vi "create default channels.vi"() -> (0 "error out":errorcluster, 1 "names":string[](array[string]), 2 "channels":refnum<class "TBM channel.lvclass">[](array[class]), 3 "module":refnum<class "UI Reference configuration.lvclass">, 5 "instance identifier":string)   [LabVIEW 2013, in "UI reference module tests.lvlib"]
uses:
  UI reference module tests.lvlib
  <vilib>/NI/Tag Bus Module Framework/channel/TBM channel.lvclass
  module/configuration/UI Reference configuration.lvclass
  <vilib>/NI/Tag Bus Module Framework/channel/channel classification.ctl
  module/configuration/UI Reference configuration.lvclass/UI Reference configuration.ctl
  module/configuration/Write VI name.vi
  module/configuration/Write VI Refnum.vi
  <vilib>/NI/Tag Bus Module Framework/root configuration/TBM configuration.lvclass
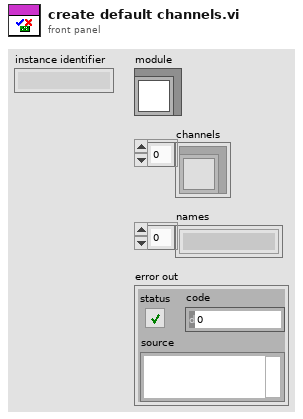
[diagram p1: front panel]
types:
  T1 = typedef "TBM channel.lvclass/channel classification.ctl" = enum16{"input data", "output data", "processing parameter", "processing result"}
  T2 = typedef "tag bus.lvlib/tag descriptor.lvclass/Data Type.ctl" = enum16{"Double", "Single", "I64", "I32", "I16", "I8", "U64", "U32", "U16", "U8", "Boolean", "String", "Array of Double", "Array of Single", "Array of I64", "Array of I32", "Array of I16", "Array of I8", "Array of U64", "Array of U32", "Array of U16", "Array of U8", "Array of Boolean", "Array of String"}
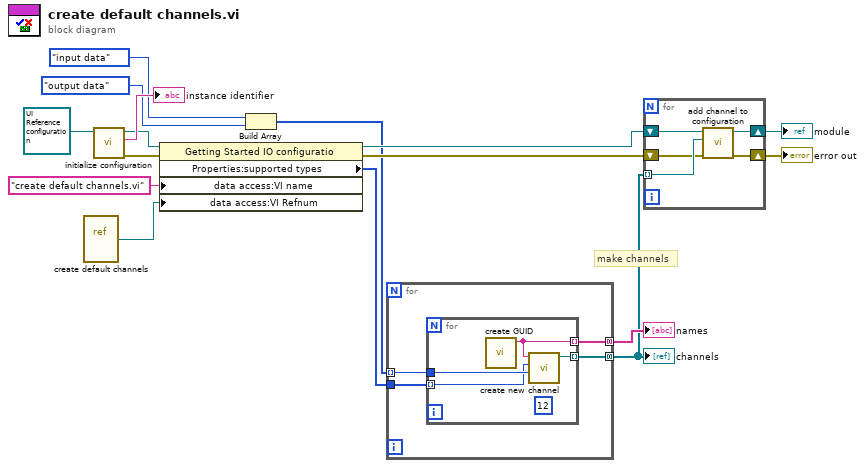
[diagram p0: block diagram]
diagram:
  # "make channels"
  n1 = vi-ref "create default channels.vi"() -> (w1:refnum<vi>)
  n2 = call-dynamic "initialize configuration.vi"("configuration in"=refnum<class "UI Reference configuration.lvclass"> refnum ("tag bus configurable plugin module configuration")) -> ("error out"=w14:errorcluster, "instance identifier"=→"instance identifier":string, "configuration out"=w11:refnum<class "UI Reference configuration.lvclass">)  [unwired: 8 in]
  n3 = property class="Getting Started IO configuratio"(reference=w11, error in=w14, "data access:VI name"="create default channels.vi" ("VI name"), "data access:VI Refnum"=w1) -> (reference out=w6:refnum<class "UI Reference configuration.lvclass">, error out=w13:errorcluster, "Properties:supported types"=w7:T2[])
  n4 = Build Array(channel_classification."input data" ("channel classification"), channel_classification."output data" ("channel classification")) -> (w5:T1[])
  n5 = for {
    tunnel: w5 -> [w20] mode=indexing
    tunnel: [w18] -> w10 mode=concatenating
    tunnel: w7 -> [w19]
    tunnel: [w17] -> w12 mode=concatenating
    n6 = for {
      tunnel: w20 -> [w23]
      tunnel: [w24] -> w18 mode=indexing
      tunnel: w19 -> [w22] mode=indexing
      tunnel: [w21] -> w17 mode=indexing
      (unwired) 12
      n7 = call <vilib>:"create GUID.vi"() -> ("uuid"=w21:string)  [unwired: 11 in]
      n8 = call <vilib>:"create new channel.vi"("channel classification"=w23, "data type"=w22, "channel name"=w21) -> ("channel"=w24:refnum<class "TBM channel.lvclass">)  [unwired: 8 in]
    }
  }
  "names" <- w12
  "channels" <- w10
  n9 = for {
    tunnel: w10 -> [w27] mode=indexing
    shift-right: [w28] -> w9
    shift-left: w6 -> [w29]
    shift-right: [w25] -> w16
    shift-left: w13 -> [w26]
    n10 = call "add channel to configuration.vi"("error in"=w26, "channel"=w27, "Getting Started IO configuration in"=w29) -> ("error out"=w25:errorcluster, "Getting Started IO configuration out"=w28:refnum<class "UI Reference configuration.lvclass">)  [unwired: 7 in]
  }
  "error out" <- w16
  "module" <- w9
